vi "GLdrv_COMMON_SAV.vi"(0 "Connection ID":T1, 11 "error in (no error)":errorcluster) -> (4 "Connection ID Out":T1, 15 "error out":errorcluster)   [LabVIEW 2017, in "GL860_Driver.lvlib"]
doc: "I/Fコマンドから記録計本体の設定を変更した場合、設定は保存\nされません。記録計本体の電源Off時にクリアされてしまいま\nす。I/Fコマンドからの設定状態を記録計本体に保存するには本\nコマンドを送信してください。\n※本コマンドは記録計本体内の設定記憶チップへの書き込みを行い\nます。本コマンドを頻繁に発行すると、設定記憶チップの寿命が短くな\nりますので、頻繁に発行する事は控えてください。"
uses:
  GL860_Driver.lvlib
  ConnectionID.ctl
  GLdrv_RW.ctl
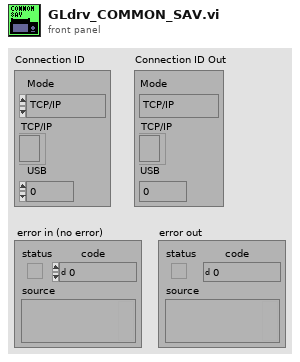
[diagram p1: front panel]
types:
  T1 = typedef "ConnectionID.ctl" = cluster{"Mode":enum16{"TCP/IP", "USB"}, "TCP/IP":refnum<k5>, "USB":i32}
  T2 = typedef "GLdrv_RW.ctl" = enum16{"Auto", "Read", "Write", "Buffer"}
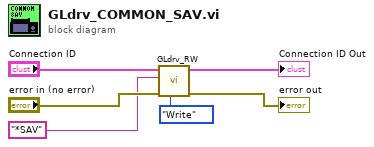
[diagram p0: block diagram]
diagram:
  n1 = call "GLdrv_RW.vi"("Mode(read)"=GLdrv_RW."Write", "error in (no error)"="error in (no error)", "data in"="*SAV" ("Command"), "Connection ID"="Connection ID") -> ("error out"=→"error out":errorcluster, "Connection ID Out"=→"Connection ID Out":T1)  [unwired: 3 in, 3 out]
